vi "test_Rx Exec Unit (Monitor).vi"() -> ()   [LabVIEW 2020]
uses:
  Shared/hardware_channels_rx.ctl
  Shared/channel_settings_rx.ctl
  <instrlib>/AIM GmbH/_AIM 664/_controls/session_monitor_config.ctl
  Shared/monitor_queue_settings.ctl
  Shared/loggingThreshold_types.ctl
  Engine/Interfaces/Shared Resources/Shared Resources.lvclass
  <vilib>/NI VeriStand/Custom Device API/Custom Device Item Ref.ctl
  Engine/Implementation/Monitor Execution Unit/Monitor Execution Unit.lvclass
  <vilib>/NI VeriStand/Custom Device API/Custom Device API.lvlib
  <instrlib>/AIM GmbH/_AIM 664/AIM664LV.lvlib
panel:
  in  "Activate Logging?":bool=TRUE
  out "?":string[](array[string])=["QueueStatus", "FramesToRead", "BytesToRead", "RxStatus", "TotalByteCount", "FrameGoodCount", "FrameErrorCount", "BytesPerSecond", "FramesPerSecond", "PhysErrorCount", "PreamErrorCount", "UnaligErrorCount", "CRCErrorCount", "IFGErrorCount", "IPErrorCount", "MACErrorCount", "NoSfdErrorCount", "VLLenErrorCount", "SNIntegrityErrorCount", "TrafShapingViolationCount", "MAC1Short", "MAC64To127Count", "MAC128To255Count", "MAC256To511Count", "MAC512To1023Count", "MAC1024To1518Count", "MACLong"]
  in  "Log Enable":bool
  out "exec time us":u32(graph)
  in  "value":T1={"channel #"=0, "channel handle"=0, "InstrumentHandle_board"=0, "InstrumentHandle_port"=0, "Queue ID"=0, "channel settings"={"Monitor Settings"={"DefaultCronoMode"=1, "GlbMonBufferSizeIn"=0}, "Rx Board"=1, "Rx Port"=0}, "current log file name"=path "", "monitor queue settings"={"TriggerPosition"=0, "CaptureMode"=1, "Strobe"=0, "MaxFileSize MB (1)"=0}, "Log File Directory"="/home/lvuser", "Base name"="test1.pcap", "Timestamp"=TRUE, "log thresholds"={"Segmentation Threshold"=1.0, "Disk Space Percentage"=5.0, "Check Disk Space"=FALSE, "Segment File"=FALSE, "Segment Files By"=0}} {"log thresholds"."Segment Files By" items=["Time", "Size"]; "monitor queue settings"."Strobe" items=["FDX_MON_STROBE_DIS", "FDX_MON_STROBE_STOP", "FDX_MON_STROBE_START"]; "monitor queue settings"."CaptureMode" items=["FDX_MON_SINGLE ", "FDX_MON_CONTINUOUS", "FDX_MON_SELECTIVE", "FDX_MON_RECORDING", "FDX_MON_REROS", "FDX_MON_HMU"]; "channel settings"."Monitor Settings"."DefaultCronoMode" items=["FDX_RX_DEFAULT_ENA_CNT", "FDX_RX_DEFAULT_MON_ENA_ALL", "FDX_RX_DEFAULT_MON_ENA_GOOD"]}
  out "Values out":dbl[](array[numeric])
  out "error out":errorcluster
  in  "stop":bool
  in  "loop rate mS":u32=10
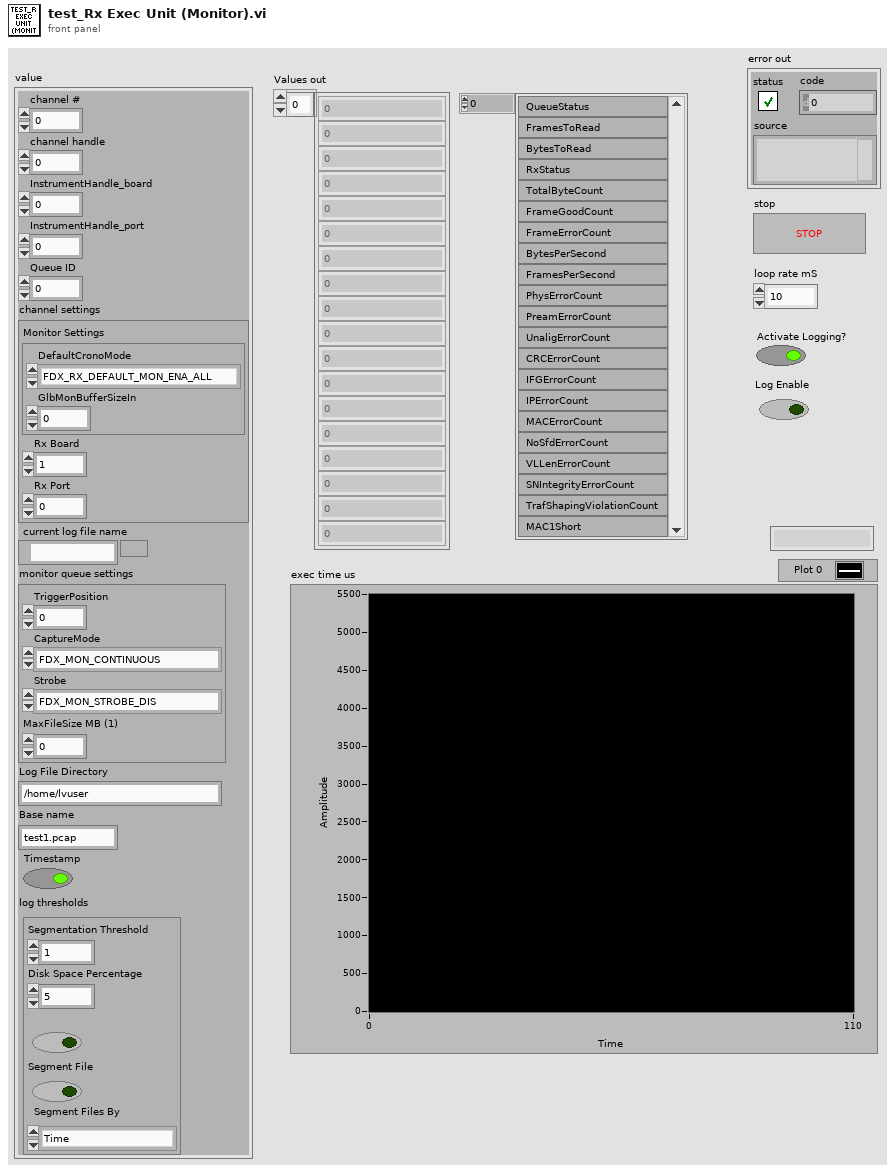
[diagram p1: front panel]
types:
  T1 = typedef "hardware_channels_rx.ctl" = cluster{"channel #":u16, "channel handle":u64, "InstrumentHandle_board":u32, "InstrumentHandle_port":u32, "Queue ID":u32, "channel settings":T2, "current log file name":path, "monitor queue settings":T4, "Log File Directory":string, "Base name":string, "Timestamp":bool, "log thresholds":T5}
  T2 = typedef "channel_settings_rx.ctl" = cluster{"Monitor Settings":T3, "Rx Board":u32, "Rx Port":u32}
  T3 = typedef "AIM664LV.lvlib/session_monitor_config.ctl" = cluster{"DefaultCronoMode":u32, "GlbMonBufferSizeIn":u32}
  T4 = typedef "monitor_queue_settings.ctl" = cluster{"TriggerPosition":u32, "CaptureMode":u32, "Strobe":u32, "MaxFileSize MB (1)":u32}
  T5 = typedef "loggingThreshold_types.ctl" = cluster{"Segmentation Threshold":dbl, "Disk Space Percentage":dbl, "Check Disk Space":bool, "Segment File":bool, "Segment Files By":u16}
  T6 = typedef "Custom Device API.lvlib/Custom Device Item Ref.ctl" = u64
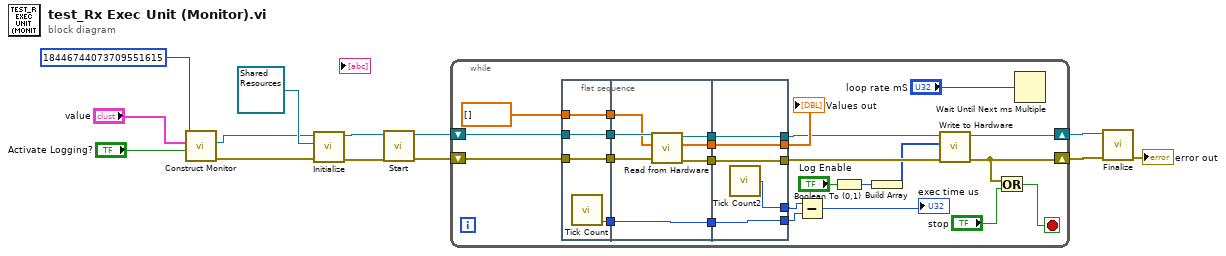
[diagram p0: block diagram]
diagram:
  n1 = call "Construct Monitor.vi"("Enable Logging?"="Activate Logging?", "Monitor Parameters"="value", "custom device ref in"=T6 18446744073709551615) -> ("error out"=w5:errorcluster, "Monitor Execution Unit out"=w3:refnum<class "Monitor Execution Unit.lvclass">)  [unwired: 5 in, 1 out]
  n2 = call-dynamic "Initialize.vi"("error in"=w5, "shared resources"=refnum<class "Shared Resources.lvclass"> refnum, "Monitor Execution Unit Implementation in"=w3) -> ("error out"=w8:errorcluster, "Monitor Execution Unit Implementation out"=w13:refnum<class "Monitor Execution Unit.lvclass">)  [unwired: 7 in]
  n3 = call-dynamic "Start.vi"("error in"=w8, "Monitor Execution Unit Implementation in"=w13) -> ("error out"=w11:errorcluster, "Monitor Execution Unit Implementation out"=w12:refnum<class "Monitor Execution Unit.lvclass">)  [unwired: 8 in]
  n4 = while {
    shift-right: [w18] -> w10
    shift-left: w12 -> [w38]
    shift-right: [w17] -> w9
    shift-left: w11 -> [w37]
    stop <- w34 stop-if-true
    n5 = flat-sequence {
      tunnel: dbl[] [] ("Values in") -> [w40]
      tunnel: w37 -> [w41]
      tunnel: w38 -> [w42]
      tunnel: [w42] -> w28
      tunnel: [w41] -> w27
      tunnel: [w40] -> w26
      tunnel: [w39] -> w24
      tunnel: [w47] -> w31
      tunnel: [w46] -> w30
      tunnel: [w45] -> w29
      tunnel: w28 -> [w49]
      tunnel: w27 -> [w48]
      tunnel: w26 -> [w44]
      tunnel: [w43] -> w25
      tunnel: w24 -> [w43]
      tunnel: [w52] -> w33
      tunnel: [w53] -> w19
      tunnel: [w54] -> w20
      tunnel: w31 -> [w54]
      tunnel: w30 -> [w53]
      tunnel: w29 -> [w52]
      tunnel: [w51] -> w23
      tunnel: w25 -> [w51]
      tunnel: [w50] -> w22
      frame #0 {
        n6 = call "Tick Count"() -> ("Tick Count(uSec)"=w39:u32)
      }
      frame #1 {
        n7 = call-dynamic "Read from Hardware.vi"("error in"=w48, "Values in"=w44, "Monitor Execution Unit Implementation in"=w49) -> ("error out"=w46:errorcluster, "Values out"=w45:dbl[], "Monitor Execution Unit Implementation out"=w47:refnum<class "Monitor Execution Unit.lvclass">)  [unwired: 6 in]
      }
      frame #2 {
        n8 = call "Tick Count2"() -> ("Tick Count(uSec)"=w50:u32)
      }
    }
    n9 = Subtract(x=w22, y=w23) -> (x-y=→"exec time us":u32)
    n10 = Boolean To (0,1)(Boolean="Log Enable") -> (0, 1=w15:i16)
    n11 = Build Array(w15) -> (w14:i16[])
    n12 = call-dynamic "Write to Hardware.vi"("error in (no error)"=w19, "Values in"=w14, "Monitor Execution Unit Implementation in"=w20) -> ("error out"=w17:errorcluster, "Monitor Execution Unit Implementation out"=w18:refnum<class "Monitor Execution Unit.lvclass">)  [unwired: 5 in, 2 out]
    n13 = Or(x=w17, y="stop") -> (x .or. y?=w34:bool)
    n14 = Wait Until Next ms Multiple(millisecond multiple="loop rate mS") -> ()  [unwired: 1 out]
    "Values out" <- w33
  }
  n15 = call-dynamic "Finalize.vi"("error in"=w9, "Monitor Execution Unit in"=w10) -> ("error out"=→"error out":errorcluster)  [unwired: 8 in, 1 out]
